vi "Datalogging.vi"   [LabVIEW 2018]
uses:
  <vilib>/Rock Robotics/WPI/ThirdParty/Phoenix-LabVIEW/Motor Controller/Get/CTRE_Phoenix_MotorController_GetQuadratureData.vi
  Robot Global Data.vi
  <vilib>/Utility/file.llb/Write Delimited Spreadsheet (string).vi
types:
  T1 = typedef "WPI_MotorControlDeviceRef.ctl" = cluster{"DeviceStatus":errorcluster, "Type":T2, "PWM":cluster{"PWM Channel":T3, "DeadBand":T4}, "CAN":cluster{"Device Number":u8, "SetOutput VI Ref":variant, "GetOutput VI Ref":variant, "Enable VI Ref":variant, "Disable VI Ref":variant, "Data":variant}, "Invert":bool, "DIO PWM":cluster{"PWM \"Enable\" Channel":T3, "DIOChannel":T5, "PWM Rate":dbl}}
  T2 = typedef "WPI_MotorControlType.ctl" = enum16{"PWM", "CAN", "DIO PWM"}
  T3 = typedef "FPGA_DIOPWMChannel.ctl" = enum8{"PWM 0", "PWM 1", "PWM 2", "PWM 3", "PWM 4", "PWM 5", "PWM 6", "PWM 7", "PWM 8", "PWM 9", "PWM MXP 0", "PWM MXP 1", "PWM MXP 2", "PWM MXP 3", "PWM MXP 4", "PWM MXP 5", "PWM MXP 6", "PWM MXP 7", "PWM MXP 8", "PWM MXP 9", "Invalid"}
  T4 = typedef "WPI_PWMDeadband.ctl" = cluster{"Name":string, "maxPositivePwm":i32, "minPositivePwm":i32, "centerPwm":i32, "maxNegativePwm":i32, "minNegativePwm":i32, "angularRange":u16}
  T5 = typedef "FPGA_DIOChannel.ctl" = enum8{"DIO 0", "DIO 1", "DIO 2", "DIO 3", "DIO 4", "DIO 5", "DIO 6", "DIO 7", "DIO 8", "DIO 9", "DIO MXP 0", "DIO MXP 1", "DIO MXP 2", "DIO MXP 3", "DIO MXP 4", "DIO MXP 5", "DIO MXP 6", "DIO MXP 7", "DIO MXP 8", "DIO MXP 9", "DIO MXP 10", "DIO MXP 11", "DIO MXP 12", "DIO MXP 13", "DIO MXP 14", "DIO MXP 15", "SPI Port CS1", "SPI Port CS2", "SPI Port CS3", "SPI Port MISO", "SPI Port MOSI", "Invalid"}
  T6 = cluster{"Yaw":dbl, "Roll":dbl, "Pitch":dbl, "Heading":dbl, "Fused Heading":dbl}
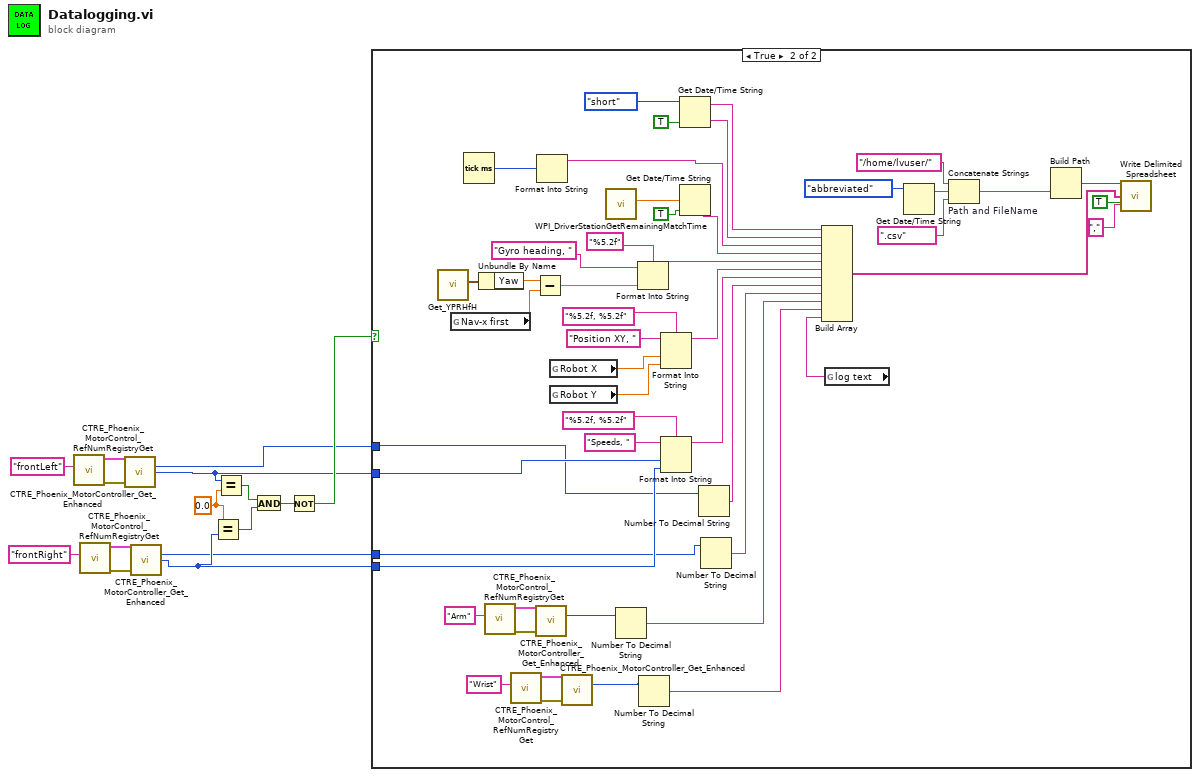
[diagram p0: block diagram]
diagram:
  w15 = 0.0 ("y")
  n1 = call <vilib>:"CTRE_Phoenix_MotorControl_RefNumRegistryGet.vi"("refnum name"="frontLeft") -> ("error out"=w10:errorcluster, "PhoenixMotorControlDevRef"=w9:T1)  [unwired: 9 in]
  n2 = call <vilib>:"CTRE_Phoenix_MotorControl_RefNumRegistryGet.vi"("refnum name"="frontRight") -> ("error out"=w6:errorcluster, "PhoenixMotorControlDevRef"=w5:T1)  [unwired: 9 in]
  n3 = call-poly <vilib>:"CTRE_Phoenix_MotorController_Get_Enhanced.vi"("PhoenixMotorControlDevRef"=w9, "error in"=w10) -> ("Quadrature Position"=w2:i32, "Quadrature Velocity"=w7:i32)  [unwired: 10 in, 2 out]
  n4 = call-poly <vilib>:"CTRE_Phoenix_MotorController_Get_Enhanced.vi"("PhoenixMotorControlDevRef"=w5, "error in"=w6) -> ("Quadrature Position"=w1:i32, "Quadrature Velocity"=w3:i32)  [unwired: 10 in, 2 out]
  n5 = Equal?(x=w15, y=w3) -> (x = y?=w13:bool)
  n6 = Equal?(x=w7, y=w15) -> (x = y?=w14:bool)
  n7 = And(x=w14, y=w13) -> (x .and. y?=w12:bool)
  n8 = Not(x=w12) -> (.not. x?=w11:bool)
  n9 = case shown="True" w11 {
    tunnel: w7 -> [_ w32]
    tunnel: w3 -> [_ w31]
    tunnel: w2 -> [_ w30]
    tunnel: w1 -> [_ w29]
    frame False {
    }
    frame True {
      n10 = call <vilib>:"Get_YPRHfH.vi"() -> ("YRPHfH"=w57:T6)  [unwired: 11 in]
      n11 = global read "Robot Global Data.vi" "Nav-x first"() -> (w65:dbl)
      n12 = Tick Count (ms)() -> (millisecond timer value=w34:u32)
      n13 = Unbundle By Name(w57) -> ("Yaw"=w58:dbl)
      n14 = call <vilib>:"CTRE_Phoenix_MotorControl_RefNumRegistryGet.vi"("refnum name"="Arm") -> ("error out"=w22:errorcluster, "PhoenixMotorControlDevRef"=w23:T1)  [unwired: 9 in]
      n15 = call <vilib>:"CTRE_Phoenix_MotorControl_RefNumRegistryGet.vi"("refnum name"="Wrist") -> ("error out"=w25:errorcluster, "PhoenixMotorControlDevRef"=w26:T1)  [unwired: 9 in]
      n16 = Subtract(x=w58, y=w65) -> (x-y=w55:dbl)
      n17 = call-poly <vilib>:"CTRE_Phoenix_MotorController_Get_Enhanced.vi"("PhoenixMotorControlDevRef"=w23, "error in"=w22) -> ("Quadrature Position"=w19:i32)  [unwired: 10 in, 3 out]
      n18 = Format Into String(w34) -> (resulting string=w33:string)  [unwired: 3 in, 1 out]
      n19 = global read "Robot Global Data.vi" "Robot X"() -> (w48:dbl)
      n20 = global read "Robot Global Data.vi" "Robot Y"() -> (w40:dbl)
      n21 = call-poly <vilib>:"CTRE_Phoenix_MotorController_Get_Enhanced.vi"("PhoenixMotorControlDevRef"=w26, "error in"=w25) -> ("Quadrature Position"=w20:i32)  [unwired: 10 in, 3 out]
      n22 = call <vilib>:"WPI_DriverStationGetRemainingMatchTime.vi"() -> ("Match Time(s)"=w64:sgl)  [unwired: 10 in, 1 out]
      n23 = Number To Decimal String(number=w19) -> (decimal integer string=w18:string)  [unwired: 1 in]
      n24 = Format Into String(format string="%5.2f", initial string="Gyro heading, " ("element"), w55) -> (resulting string=w37:string)  [unwired: 1 in, 1 out]
      n25 = Number To Decimal String(number=w20) -> (decimal integer string=w17:string)  [unwired: 1 in]
      n26 = Format Into String(format string="%5.2f, %5.2f", initial string="Position XY, ", w48, w40) -> (resulting string=w36:string)  [unwired: 1 in, 1 out]
      n27 = Format Into String(format string="%5.2f, %5.2f", initial string="Speeds, ", w32, w31) -> (resulting string=w35:string)  [unwired: 1 in, 1 out]
      n28 = Get Date/Time String(date format (0)=enum16{"short", "long", "abbreviated"}."short", want seconds? (F)=TRUE) -> (date string=w47:string, time string=w46:string)  [unwired: 1 in]
      n29 = Get Date/Time String(seconds (now)=w64, want seconds? (F)=TRUE) -> (time string=w59:string)  [unwired: 1 in, 1 out]
      n30 = Number To Decimal String(number=w30) -> (decimal integer string=w28:string)  [unwired: 1 in]
      n31 = Number To Decimal String(number=w29) -> (decimal integer string=w27:string)  [unwired: 1 in]
      n32 = global read "Robot Global Data.vi" "log text"() -> (w16:string)
      n33 = Build Array(w47, w46, w33, w59, w37, w36, w35, w28, w27, w18, w17, w16) -> (w62:string[])
      n34 = Get Date/Time String(date format (0)=enum16{"short", "long", "abbreviated"}."abbreviated") -> (date string=w49:string)  [unwired: 2 in, 1 out]
      n35 = Concatenate Strings "Path and FileName"("/home/lvuser/", w49, ".csv") -> (w52:string)
      n36 = Build Path(name or relative path=w52) -> (appended path=w51:path)  [unwired: 1 in]
      n37 = call-poly <vilib>:"Write Delimited Spreadsheet.vi"("file path (dialog if empty)"=w51, "1D data"=w62, "append to file? (new file:F)"=TRUE, "delimiter (\\t)"="," ("delimiter (\\t)")) -> ()  [unwired: 10 in, 2 out]
    }
  }
